vi "StackCode.vi"   [LabVIEW 2018]
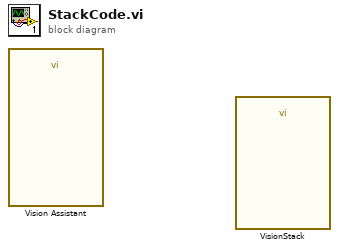
[diagram p0: block diagram]
diagram:
  n1 = call "Vision Assistant"() -> ()  [unwired: 23 in, 5 out]
  n2 = call "VisionStack"() -> ()  [unwired: 24 in, 4 out]
